vi "getAll.vi"(8 "error in (no error)":errorcluster, 11 "instrument.Cryostation in":refnum<class "instrument.Cryostation.lvclass">) -> (0 "error out":errorcluster, 2 "getAll":variant, 3 "instrument.Cryostation out":refnum<class "instrument.Cryostation.lvclass">)   [LabVIEW 2016, in "instrument.Cryostation.lvclass"]
uses:
  instrument.Cryostation.lvclass
  Typedefs/getAll--Cryostation--cluster.ctl
  instrument.Cryostation.lvclass/instrument.Cryostation.ctl
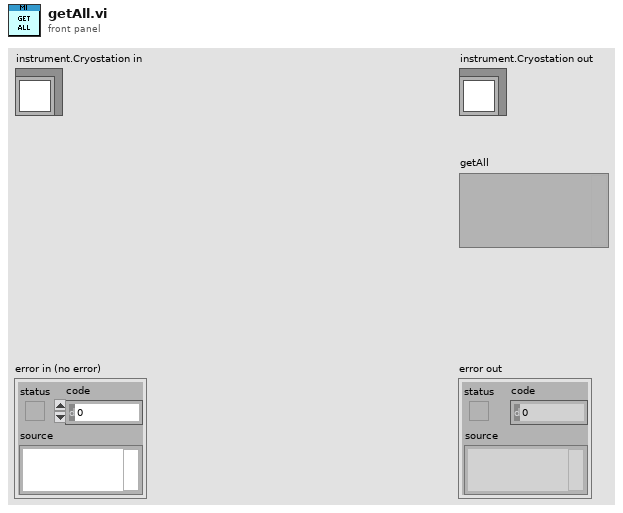
[diagram p1: front panel]
types:
  T1 = typedef "instrument.Cryostation.lvclass/getAll--Cryostation--cluster.ctl" = cluster{"Platform Temperature (K)":dbl, "Sample Temperature (K)":dbl, "Stage 1 Temperature (K)":dbl, "Stage 2 Temperature (K)":dbl, "Chamber Pressure (mTorr)":dbl}
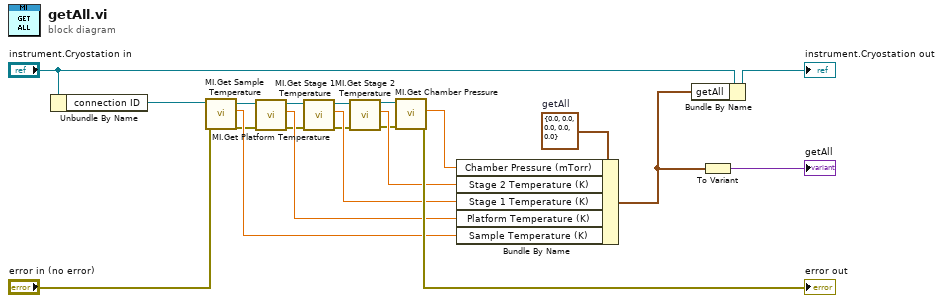
[diagram p0: block diagram]
diagram:
  w21 = T1 {"Platform Temperature (K)"=0.0, "Sample Temperature (K)"=0.0, "Stage 1 Temperature (K)"=0.0, "Stage 2 Temperature (K)"=0.0, "Chamber Pressure (mTorr)"=0.0}  # getAll
  n1 = Unbundle By Name("instrument.Cryostation in") -> ("connection ID"=w19:refnum<k5>)
  n2 = call "MI.Get Sample Temperature.vi"("error in (no error)"="error in (no error)", "TCP Network Connection in"=w19) -> ("error out"=w7:errorcluster, "Sample Temperature (K)"=w9:dbl, "TCP Network Connection out"=w8:refnum<k5>)  [unwired: 7 in]
  n3 = call "MI.Get Platform Temperature.vi"("error in (no error)"=w7, "TCP Network Connection in"=w8) -> ("error out"=w5:errorcluster, "Platform Temperature (K)"=w10:dbl, "TCP Network Connection out"=w6:refnum<k5>)  [unwired: 7 in]
  n4 = call "MI.Get Stage 1 Temperature.vi"("error in (no error)"=w5, "TCP Network Connection in"=w6) -> ("error out"=w3:errorcluster, "Stage 1 Temperature (K)"=w11:dbl, "TCP Network Connection out"=w4:refnum<k5>)  [unwired: 7 in]
  n5 = call "MI.Get Stage 2 Temperature.vi"("error in (no error)"=w3, "TCP Network Connection in"=w4) -> ("error out"=w1:errorcluster, "Stage 2 Temperature (K)"=w12:dbl, "TCP Network Connection out"=w2:refnum<k5>)  [unwired: 7 in]
  n6 = call "MI.Get Chamber Pressure.vi"("error in (no error)"=w1, "TCP Network Connection in"=w2) -> ("error out"=→"error out":errorcluster, "Chamber Pressure (mTorr)"=w13:dbl)  [unwired: 7 in, 1 out]
  n7 = Bundle By Name(cluster=w21, "Chamber Pressure (mTorr)"=w13, "Stage 2 Temperature (K)"=w12, "Stage 1 Temperature (K)"=w11, "Platform Temperature (K)"=w10, "Sample Temperature (K)"=w9) -> (w15:T1)
  n8 = Bundle By Name(cluster="instrument.Cryostation in", "getAll"=w15) -> (→"instrument.Cryostation out":refnum<class "instrument.Cryostation.lvclass">)
  n9 = To Variant(anything=w15) -> (Variant=→"getAll":variant)
